vi "rad_Load Targets from File.vi"(11 "PathFile":path) -> (1 "Valid File":bool, 3 "IPs to Load":string[](array[string]))   [LabVIEW 2020]
doc: "Opens the provided txt file and returns a list with the IP Addresses found. IPs are expected to be in the format xx.xx.xx.xx. IPs with different format will be filtered. s"
uses:
  <vilib>/Utility/file.llb/Read From Spreadsheet File (string).vi
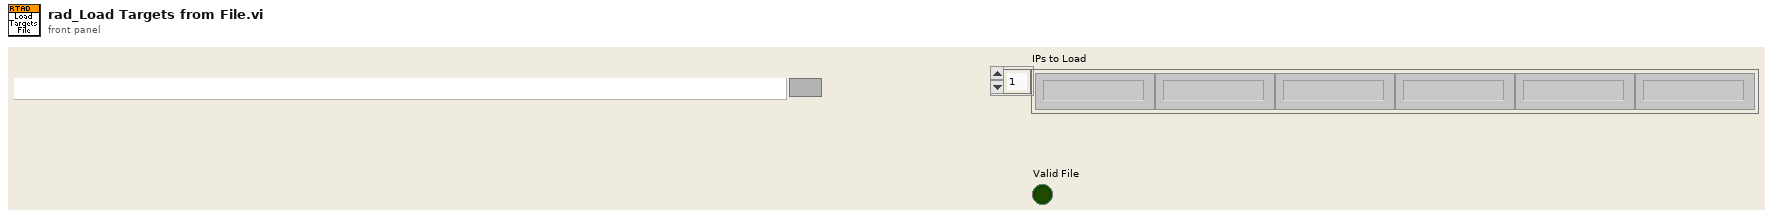
[diagram p1: front panel]
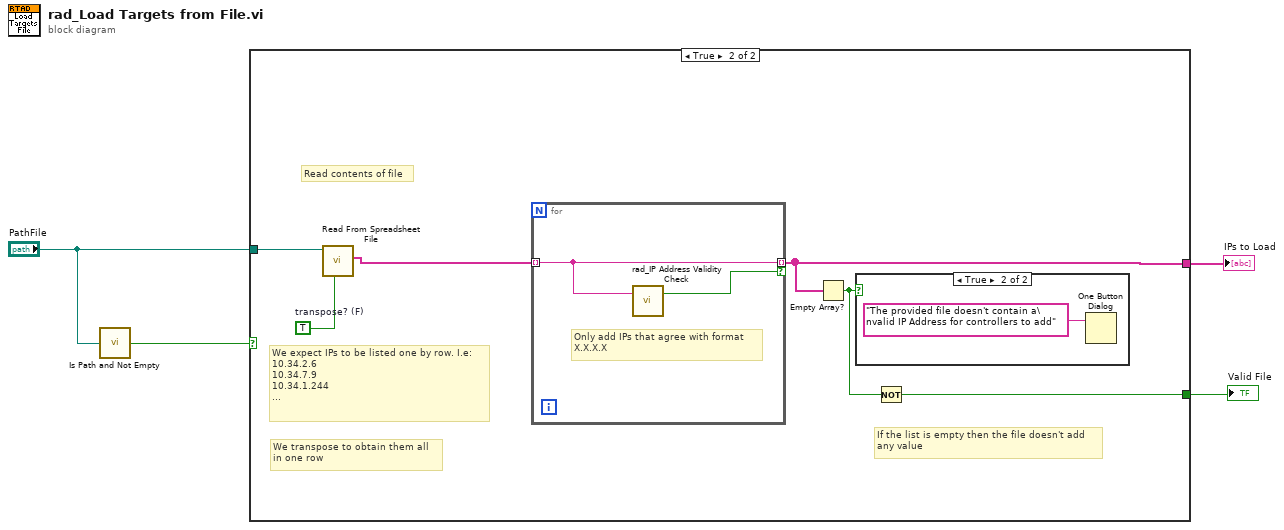
[diagram p0: block diagram]
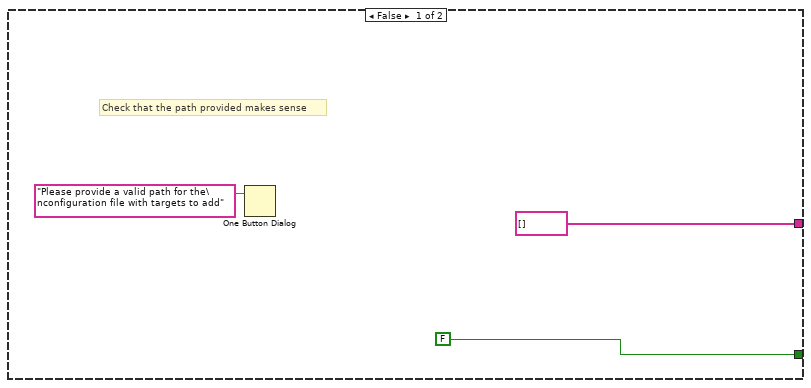
[diagram p2: hidden frame]
diagram:
  n1 = call <vilib>:"Is Path and Not Empty.vi"("path"="PathFile") -> ("Is Path and Not Empty?"=w3:bool)  [unwired: 4 in]
  n2 = case shown="True" w3 {
    tunnel: "PathFile" -> [_ w13]
    tunnel: [FALSE w11] -> w2
    tunnel: [string[] [] w10] -> w1
    frame False {
      # "Check that the path provided makes sense"
      n3 = One Button Dialog(message="Please provide a valid path for the\nconfiguration file with targets to add") -> ()  [unwired: 1 in, 1 out]
    }
    frame True {
      w12 = TRUE  # transpose? (F)
      # "If the list is empty then the file doesn't add\nany value"
      # "We transpose to obtain them all\nin one row"
      # "We expect IPs to be listed one by row. I.e:\n10.34.2.6\n10.34.7.9\n10.34.1.244\n..."
      # "Read contents of file"
      n4 = call-poly <vilib>:"Read From Spreadsheet File.vi"("transpose (no:F)"=w12, "file path (dialog if empty)"=w13) -> ("first row"=w8:string[])  [unwired: 5 in, 4 out]
      n5 = for {
        tunnel: w8 -> [w16] mode=indexing
        tunnel: [w16] -> w10 mode=indexing if=w15
        # "Only add IPs that agree with format\nX.X.X.X"
        n6 = call "rad_IP Address Validity Check.vi"("IP Address"=w16) -> ("Valid IP"=w15:bool)  [unwired: 2 in]
      }
      n7 = Empty Array?(array=w10) -> (empty?=w9:bool)
      n8 = case shown="True" w9 {
        frame False {
        }
        frame True {
          n9 = One Button Dialog(message="The provided file doesn't contain a\nvalid IP Address for controllers to add") -> ()  [unwired: 1 in, 1 out]
        }
      }
      n10 = Not(x=w9) -> (.not. x?=w11:bool)
    }
  }
  "IPs to Load" <- w1
  "Valid File" <- w2
